vi "TRR_Main.vi"() -> ()   [LabVIEW 2020]
uses:
  Global 1.vi
panel:
  in  "Median Filter Rank":i32=5
  out "CURRENT RESULT":dbl[](array[numeric])
  in  "START TEST":bool
  out "Started":bool
  out "Elapsed time (minutes)":dbl
  out "start time":timestamp
  out "Oscilloscope Capture":waveform(dbl)[](graph)
  out "ALL RESULT Array":dbl[][](array[numeric])
  out "TEST#   |  Elapsed Time (minutes)":dbl[][](array[numeric])
  out "TRR :\nTotal Test Time (minutes)":dbl
  in  "Finish?":bool
  out "Cluster 3":T1
  out "Cluster 2":T2
  out "Cluster 1":T3
  in  "Cluster : Setting":T4={"VGE (V)"=0.0, "VCE (V)"=0.0, "ICE (A)"=0.0, "TEKTRONIX"="", "PROJECT #"="", "TEMPERATURE (C)"=0.0, "RG (Ohm)"=0.0, "DUT #"=1, "REQUEST #"="", "TEST #"=1}
  out "error out":errorcluster
  in  "error in (no error)":errorcluster
  # "PRODUCED BY : AFIQAH HASBULLAH ( SBN CZ ENG : 2022)"
  # "AC MODULE : TRR"
  # "Column 2"
  # "Column 3"
  # "Column 4"
  # "Column 5"
  # "Column 6"
  # "Column 7"
  # "Column 8"
  # "Column 9"
  # "Column 10"
  # "Column 0"
  # "Column 1"
  # "Column 11"
  # "Column 12"
  # "Column 13"
  # "Column 14"
  # "Column 15"
  # "Ta\n(ns)"
  # "Tb\n(ns)"
  # "Trr\n(ns)"
  # "Irrm\n(A)"
  # "Qrr\n(nC)"
  # "Erec\n(uJ)"
  # "Di/Dt\n(A/us)"
  # "Di\n(A)"
  # "Dt\n(us)"
  # "Vce"
  # "Ice"
  # "Vge"
  # "Rg"
  # "Temperature"
  # "DUT  #"
  # "TEST #"
  # "< Press 2 times >"
  # "Column 2"
  # "Column 3"
  # "Column 4"
  # "Column 5"
  # "Column 6"
  # "Column 7"
  # "Column 8"
  # "Column 9"
  # "Column 10"
  # "Column 0"
  # "Column 1"
  # "Column 11"
  # "Column 12"
  # "Column 13"
  # "Column 14"
  # "Column 15"
  # "Ta\n(ns)"
  # "Tb\n(ns)"
  # "Trr\n(ns)"
  # "Irrm\n(A)"
  # "Qrr\n(nC)"
  # "Erec\n(uJ)"
  # "Di/Dt\n(A/us)"
  # "Di\n(A)"
  # "Dt\n(us)"
  # "Vce"
  # "Ice"
  # "Vge"
  # "Rg"
  # "Temperature"
  # "DUT  #"
  # "TEST #"
  # "Done TRR & QRR Acquisition"
  # "Done Di/Dt Acquisition"
  # "Done Exporting image of Overall Waveform"
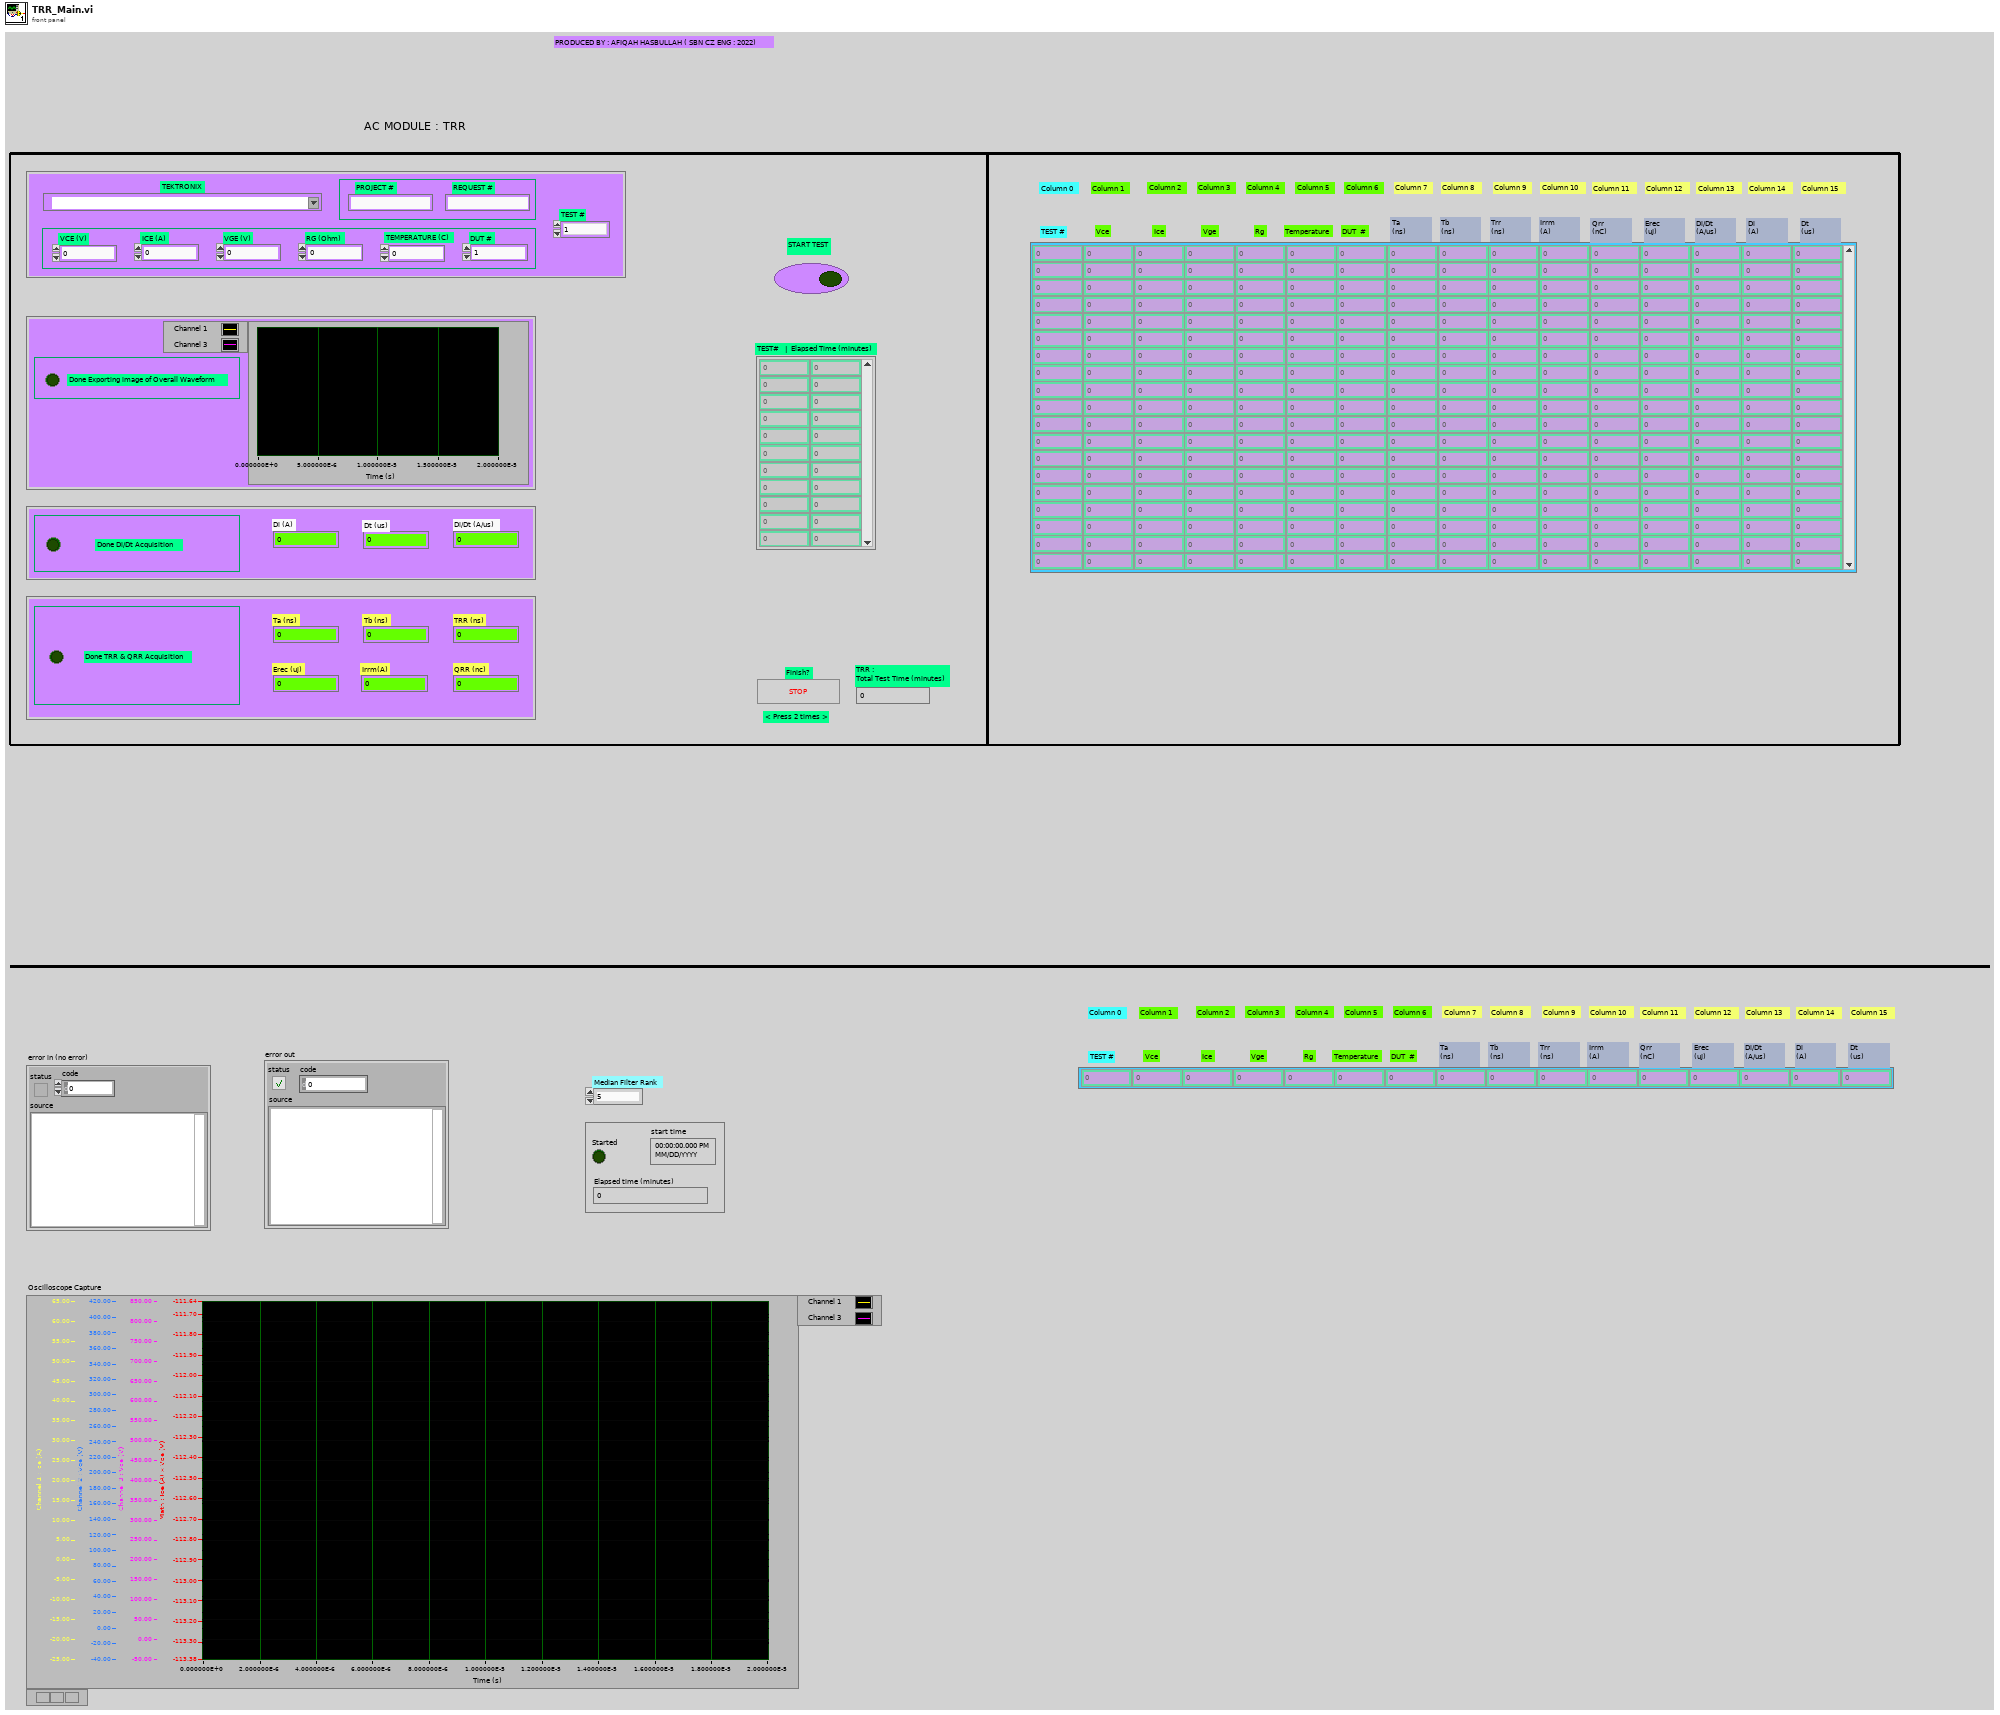
[diagram p1: front panel]
types:
  T1 = cluster{"Ta (ns)":dbl, "Tb (ns)":dbl, "Irrm(A)":dbl, "TRR (ns)":dbl, "QRR (nc)":dbl, "Erec (uj)":dbl, "LED 3":bool}
  T2 = cluster{"Di/Dt (A/us)":dbl, "Di (A)":dbl, "Dt (us)":dbl, "LED 2":bool}
  T3 = cluster{"LED 1":bool, "Oscilloscope Capture":waveform(dbl)[]}
  T4 = cluster{"VGE (V)":dbl, "VCE (V)":dbl, "ICE (A)":dbl, "TEKTRONIX":refnum<visa-resource-name>, "PROJECT #":string, "TEMPERATURE (C)":dbl, "RG (Ohm)":dbl, "DUT #":i32, "REQUEST #":string, "TEST #":i32}
  T5 = cluster{"Di/Dt (A/us)":dbl, "Di (A)":dbl, "Dt (ns)":dbl, "LED 2":bool}
  T6 = typedef "imagedata.ctl" = cluster{"image type":i32, "image depth":i32, "image":u8[], "mask":u8[], "colors":u32[], "Rectangle":cluster{"left":i16, "top":i16, "right":i16, "bottom":i16}}
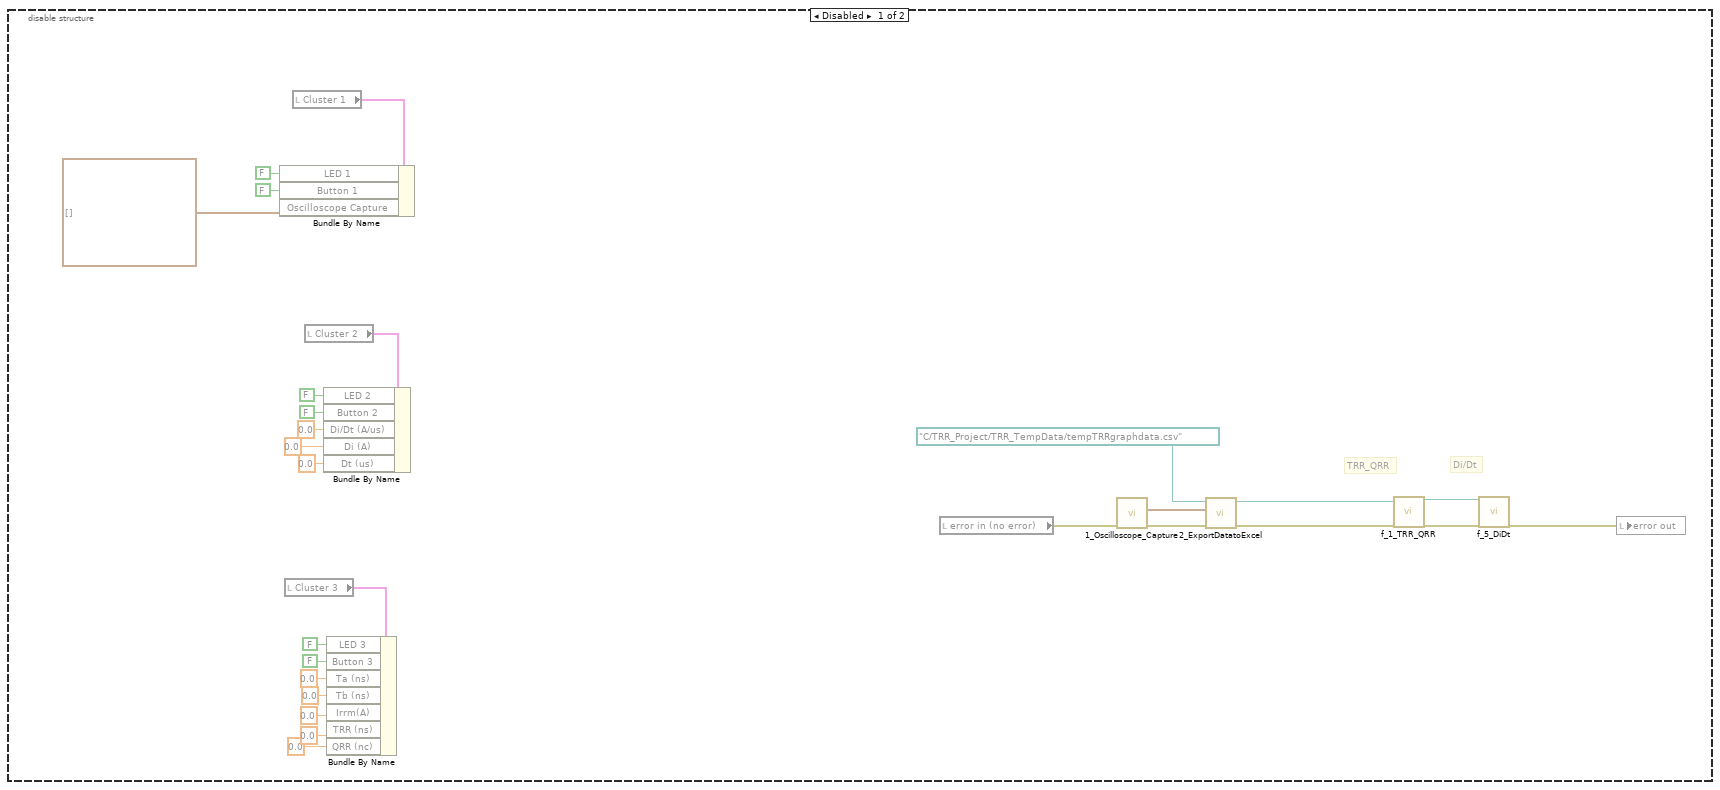
[diagram p3: hidden frame]
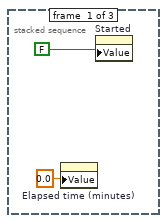
[diagram p4: hidden frame]
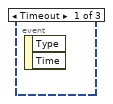
[diagram p6: hidden frame]
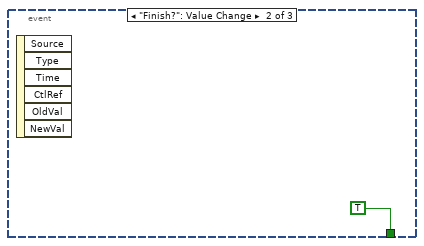
[diagram p7: hidden frame]
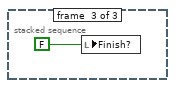
[diagram p9: hidden frame]
diagram:
  w1 = 5 ("Median Filter Rank")
  w17 = errorcluster {"status"=FALSE, "code"=0, "source"=""} ("error out")
  w4 = FALSE ("Started")
  w16 = 0.0 ("TRR :\nTotal Test Time (minutes)")
  n1 = flat-sequence {
    tunnel: [w27] -> w7
    tunnel: w7 -> [w28]
    tunnel: [w29] -> w6
    tunnel: w6 -> [w286]
    tunnel: [w281] -> w5
    tunnel: w5 -> [w312]
    frame #0 {
      # "IN"
      n2 = local read "error in (no error)"() -> (w27:errorcluster)
    }
    frame #1 {
      n3 = while {
        shift-right: [w32] -> w29
        shift-left: w28 -> [w31]
        stop <- w33 stop-if-true
        n4 = local read "START TEST"() -> (w35:bool)
        n5 = case shown="True" w35 {
          tunnel: w31 -> [w36 w53]
          tunnel: [w36 w46] -> w32
          frame False {
          }
          frame True {
            n6 = flat-sequence {
              tunnel: w53 -> [w60]
              tunnel: [w60] -> w45
              tunnel: w45 -> [w73]
              tunnel: [w73] -> w44
              tunnel: [w71] -> w43
              tunnel: [w70] -> w42
              tunnel: [w69] -> w41
              tunnel: [w68] -> w40
              tunnel: [w67] -> w39
              tunnel: [w66] -> w38
              tunnel: [w65] -> w37
              tunnel: w44 -> [w81]
              tunnel: [w81] -> w52
              tunnel: w43 -> [w80]
              tunnel: w42 -> [w79]
              tunnel: w41 -> [w78]
              tunnel: w40 -> [w77]
              tunnel: w39 -> [w76]
              tunnel: w38 -> [w75]
              tunnel: w37 -> [w74]
              tunnel: w52 -> [w108]
              tunnel: [w107] -> w51
              tunnel: w51 -> [w145]
              tunnel: [w141] -> w50
              tunnel: w50 -> [w196]
              tunnel: [w192] -> w49
              tunnel: w49 -> [w259]
              tunnel: [w259] -> w48
              tunnel: w48 -> [w267]
              tunnel: [w267] -> w47
              tunnel: w47 -> [w276]
              tunnel: [w276] -> w46
              frame #0 {
                # "Initialize"
                n7 = local read "Median Filter Rank"() -> (w54:i32)
                n8 = Initialize Array(0.0 ("element"), 16 ("dimension size")) -> (w57:dbl[])
                n9 = local write "Cluster 3"(T1 {"Ta (ns)"=0.0, "Tb (ns)"=0.0, "Irrm(A)"=0.0, "TRR (ns)"=0.0, "QRR (nc)"=0.0, "Erec (uj)"=0.0, "LED 3"=FALSE} ("Cluster 3")) -> ()
                n10 = global write "Global 1.vi" "Median Filter Rank"(w54) -> ()
                n11 = local write "Cluster 2"(T5 {"Di/Dt (A/us)"=0.0, "Di (A)"=0.0, "Dt (ns)"=0.0, "LED 2"=FALSE} ("Cluster 2")) -> ()
                n12 = local write "CURRENT RESULT"(w57) -> ()
                n13 = local write "Cluster 1"(T3 {"LED 1"=FALSE, "Oscilloscope Capture"=[]} ("Cluster 1")) -> ()
                n14 = local write "Oscilloscope Capture"(waveform(dbl)[] [] ("Oscilloscope Capture")) -> ()
                n15 = Wait (ms)(milliseconds to wait=u32 500) -> ()  [unwired: 1 out]
              }
              frame #1 {
                n16 = local read "Cluster : Setting"() -> (w72:T4)
                n17 = Unbundle By Name(w72) -> ("TEST #"=w71:i32, "VCE (V)"=w70:dbl, "ICE (A)"=w69:dbl, "VGE (V)"=w68:dbl, "RG (Ohm)"=w67:dbl, "TEMPERATURE (C)"=w66:dbl, "DUT #"=w65:i32)
                n18 = Wait (ms)(milliseconds to wait=u32 300) -> ()  [unwired: 1 out]
              }
              frame #2 {
                # "Column 6 = DUT#"
                # "Column 5 = Temperature"
                # "Column 4 = RG"
                # "Column 3 = VGE"
                # "Column 2 = ICE"
                # "Column 1 = VCE"
                # "Column 0 = TEST#"
                # "Insert Test Condition"
                n19 = Wait (ms)(milliseconds to wait=u32 300) -> ()  [unwired: 1 out]
                n20 = local read "CURRENT RESULT"() -> (w84:dbl[])
                n21 = local read "CURRENT RESULT"() -> (w86:dbl[])
                n22 = local read "CURRENT RESULT"() -> (w88:dbl[])
                n23 = local read "CURRENT RESULT"() -> (w89:dbl[])
                n24 = local read "CURRENT RESULT"() -> (w96:dbl[])
                n25 = local read "CURRENT RESULT"() -> (w92:dbl[])
                n26 = local read "CURRENT RESULT"() -> (w94:dbl[])
                n27 = Replace Array Subset(array=w96, new element=w80, index=0) -> (w95:dbl[])
                n28 = Replace Array Subset(array=w94, new element=w79, index=1) -> (w93:dbl[])
                n29 = Replace Array Subset(array=w92, new element=w78, index=2) -> (w91:dbl[])
                n30 = Replace Array Subset(array=w89, new element=w77, index=3) -> (w90:dbl[])
                n31 = Replace Array Subset(array=w84, new element=w74, index=6) -> (w83:dbl[])
                n32 = Replace Array Subset(array=w88, new element=w76, index=4) -> (w87:dbl[])
                n33 = Replace Array Subset(array=w86, new element=w75, index=5) -> (w85:dbl[])
                n34 = local write "CURRENT RESULT"(w95) -> ()
                n35 = local write "CURRENT RESULT"(w93) -> ()
                n36 = local write "CURRENT RESULT"(w91) -> ()
                n37 = local write "CURRENT RESULT"(w90) -> ()
                n38 = local write "CURRENT RESULT"(w87) -> ()
                n39 = local write "CURRENT RESULT"(w85) -> ()
                n40 = local write "CURRENT RESULT"(w83) -> ()
              }
              frame #3 {
                n41 = Wait (ms)(milliseconds to wait=u32 300) -> ()  [unwired: 1 out]
                n42 = flat-sequence {
                  tunnel: w108 -> [w115]
                  tunnel: [w110] -> w105
                  tunnel: [w120] -> w104
                  tunnel: w105 -> [w119]
                  tunnel: [w136] -> w107
                  tunnel: w104 -> [w136]
                  frame #0 {
                    n43 = local read "Cluster : Setting"() -> (w114:T4)
                    n44 = Unbundle By Name(w114) -> ("TEKTRONIX"=w113:refnum<visa-resource-name>)
                    n45 = call "1_Oscilloscope_Capture.vi"("error in (no error)"=w115, "VISA Resource Name"=w113) -> ("error out"=w111:errorcluster, "Waveform Graph"=w109:waveform(dbl)[])  [unwired: 7 in, 1 out]
                    n46 = local write "Oscilloscope Capture"(w109) -> ()
                    n47 = local read "Cluster 1"() -> (w118:T3)
                    n48 = Bundle By Name(cluster=w118, "Oscilloscope Capture"=w109) -> (w117:T3)
                    n49 = local write "Cluster 1"(w117) -> ()
                    n50 = Wait (ms)(milliseconds to wait=u32 300) -> ()  [unwired: 1 out]
                    n51 = call "2_ExportDatatoExcel.vi"("error in (no error)"=w111, "Waveform Graph"=w109, "file path (IN)"=path "C:/TRR_Project/TRR_TempData/tempFullWaveformgraphdata.csv") -> ("error out"=w110:errorcluster)  [unwired: 7 in, 1 out]
                  }
                  frame #1 {
                    w132 = "_"
                    n52 = local read "Cluster : Setting"() -> (w127:T4)
                    n53 = Unbundle By Name(w127) -> ("PROJECT #"=w124:string, "REQUEST #"=w123:string, "TEST #"=w126:i32)
                    n54 = invoke on="Oscilloscope Capture" class="WFGraph (strict)" method="Get Image"(error in=w119) -> (error out=w128:errorcluster, "image data"=w129:T6)  [unwired: 5 in, 4 out]
                    n55 = Format Value(format string="%d", value (0)=w126) -> (output string=w122:string)  [unwired: 1 in]
                    n56 = Concatenate Strings("C:\\TRR_Project\\TRR_Image\\" ("string"), w124, w132, w123, w132, w122, w132, "TRR_FullWaveform" ("string"), ".png" ("string")) -> (w135:string)
                    n57 = String To Path(string=w135) -> (path=w134:path)
                    n58 = call <vilib>:"Write PNG File.vi"("error in (no error)"=w128, "image data"=w129, "path to PNG file"=w134) -> ("error out"=w120:errorcluster)  [unwired: 7 in, 1 out]
                    n59 = Wait (ms)(milliseconds to wait=u32 300) -> ()  [unwired: 1 out]
                  }
                  frame #2 {
                    n60 = local read "Cluster 1"() -> (w140:T3)
                    n61 = Bundle By Name(cluster=w140, "LED 1"=TRUE) -> (w138:T3)
                    n62 = Wait (ms)(milliseconds to wait=u32 300) -> ()  [unwired: 1 out]
                    n63 = local write "Cluster 1"(w138) -> ()
                  }
                }
              }
              frame #4 {
                # "Step 1 : Di/Dt"
                n64 = Wait (ms)(milliseconds to wait=u32 300) -> ()  [unwired: 1 out]
                n65 = flat-sequence {
                  tunnel: w145 -> [w150]
                  tunnel: [w150] -> w144
                  tunnel: [w156] -> w149
                  tunnel: [w155] -> w148
                  tunnel: [w151] -> w147
                  tunnel: w144 -> [w153]
                  tunnel: [w152] -> w142
                  tunnel: w149 -> [w176]
                  tunnel: w148 -> [w175]
                  tunnel: w147 -> [w174]
                  tunnel: [w172] -> w143
                  tunnel: w142 -> [w172]
                  tunnel: w143 -> [w186]
                  tunnel: [w186] -> w141
                  frame #0 {
                  }
                  frame #1 {
                    # "Di/Dt"
                    n66 = local read "Cluster : Setting"() -> (w165:T4)
                    n67 = Unbundle By Name(w165) -> ("ICE (A)"=w160:dbl, "PROJECT #"=w163:string, "REQUEST #"=w162:string, "TEST #"=w166:i32, "TEKTRONIX"=w159:refnum<visa-resource-name>)
                    n68 = call "1_Oscilloscope_Capture.vi"("error in (no error)"=w153, "VISA Resource Name"=w159) -> ("error out"=w170:errorcluster, "Waveform Graph"=w171:waveform(dbl)[])  [unwired: 7 in, 1 out]
                    n69 = call "2_ExportDatatoExcel.vi"("error in (no error)"=w170, "Waveform Graph"=w171, "file path (IN)"=path "C:/TRR_Project/TRR_TempData/tempDiDtgraphdata.csv") -> ("error out"=w167:errorcluster, "file path (OUT)"=w168:path)  [unwired: 7 in]
                    n70 = Format Value(format string="%d", value (0)=w166) -> (output string=w161:string)  [unwired: 1 in]
                    n71 = call "f_5_DiDt.vi"("file path (IN)"=w168, "Project #"=w163, "Request #"=w162, "TEST #"=w161, "error in (no error)"=w167, "ICE"=w160) -> ("Dt (us)"=w151:dbl, "Di (A)"=w155:dbl, "Di/Dt (A/us)"=w156:dbl, "error out"=w152:errorcluster)  [unwired: 5 in, 5 out]
                    n72 = local read "Cluster 2"() -> (w158:T2)
                    n73 = Bundle By Name(cluster=w158, "Di/Dt (A/us)"=w156, "Di (A)"=w155, "Dt (us)"=w151) -> (w157:T2)
                    n74 = Wait (ms)(milliseconds to wait=u32 300) -> ()  [unwired: 1 out]
                    n75 = local write "Cluster 2"(w157) -> ()
                  }
                  frame #2 {
                    # "Column 15 = Dt"
                    # "Column 14 = Di"
                    # "Column 13 = DiDt"
                    n76 = local read "CURRENT RESULT"() -> (w180:dbl[])
                    n77 = local read "CURRENT RESULT"() -> (w178:dbl[])
                    n78 = local read "CURRENT RESULT"() -> (w182:dbl[])
                    n79 = Wait (ms)(milliseconds to wait=u32 300) -> ()  [unwired: 1 out]
                    n80 = Replace Array Subset(array=w178, new element=w174, index=15) -> (w177:dbl[])
                    n81 = Replace Array Subset(array=w180, new element=w175, index=14) -> (w179:dbl[])
                    n82 = Replace Array Subset(array=w182, new element=w176, index=13) -> (w181:dbl[])
                    n83 = local write "CURRENT RESULT"(w177) -> ()
                    n84 = local write "CURRENT RESULT"(w179) -> ()
                    n85 = local write "CURRENT RESULT"(w181) -> ()
                  }
                  frame #3 {
                    n86 = local read "Cluster 2"() -> (w189:T2)
                    n87 = Bundle By Name(cluster=w189, "LED 2"=TRUE ("LED 1")) -> (w190:T2)
                    n88 = Wait (ms)(milliseconds to wait=u32 300) -> ()  [unwired: 1 out]
                    n89 = local write "Cluster 2"(w190) -> ()
                  }
                }
              }
              frame #5 {
                # "Step 2 : Irrm, Ta, Tb, TRR, QRR, Erec"
                n90 = Wait (ms)(milliseconds to wait=u32 300) -> ()  [unwired: 1 out]
                n91 = flat-sequence {
                  tunnel: w196 -> [w203]
                  tunnel: [w203] -> w195
                  tunnel: [w211] -> w202
                  tunnel: [w210] -> w201
                  tunnel: [w209] -> w200
                  tunnel: [w208] -> w199
                  tunnel: [w207] -> w198
                  tunnel: [w206] -> w197
                  tunnel: w195 -> [w205]
                  tunnel: [w204] -> w193
                  tunnel: w202 -> [w234]
                  tunnel: w201 -> [w233]
                  tunnel: w200 -> [w232]
                  tunnel: w199 -> [w231]
                  tunnel: w198 -> [w230]
                  tunnel: w197 -> [w229]
                  tunnel: [w228] -> w194
                  tunnel: w193 -> [w228]
                  tunnel: w194 -> [w254]
                  tunnel: [w254] -> w192
                  frame #0 {
                  }
                  frame #1 {
                    # "TRR_QRR"
                    n92 = local read "Cluster : Setting"() -> (w223:T4)
                    n93 = Unbundle By Name(w223) -> ("ICE (A)"=w214:dbl, "PROJECT #"=w215:string, "REQUEST #"=w213:string, "TEST #"=w224:i32, "TEKTRONIX"=w221:refnum<visa-resource-name>)
                    n94 = call "1_Oscilloscope_Capture.vi"("error in (no error)"=w205, "VISA Resource Name"=w221) -> ("error out"=w226:errorcluster, "Waveform Graph"=w227:waveform(dbl)[])  [unwired: 7 in, 1 out]
                    n95 = call "2_ExportDatatoExcel.vi"("error in (no error)"=w226, "Waveform Graph"=w227, "file path (IN)"=path "C:/TRR_Project/TRR_TempData/tempTRRgraphdata.csv") -> ("error out"=w217:errorcluster, "file path (OUT)"=w216:path)  [unwired: 7 in]
                    n96 = Format Value(format string="%d", value (0)=w224) -> (output string=w212:string)  [unwired: 1 in]
                    n97 = call "f_1_TRR_QRR.vi"("file path (IN)"=w216, "Project #"=w215, "Request #"=w213, "TEST #"=w212, "error in (no error)"=w217, "ICE"=w214) -> ("Ta (ns)"=w211:dbl, "Tb (ns)"=w210:dbl, "Irrm(A)"=w208:dbl, "Erec (uj)"=w206:dbl, "TRR (ns)"=w209:dbl, "QRR (nc)"=w207:dbl, "error out"=w204:errorcluster)  [unwired: 5 in, 2 out]
                    n98 = local read "Cluster 3"() -> (w220:T1)
                    n99 = Bundle By Name(cluster=w220, "Ta (ns)"=w211, "Tb (ns)"=w210, "Irrm(A)"=w208, "TRR (ns)"=w209, "QRR (nc)"=w207, "Erec (uj)"=w206) -> (w219:T1)
                    n100 = local write "Cluster 3"(w219) -> ()
                    n101 = Wait (ms)(milliseconds to wait=u32 300) -> ()  [unwired: 1 out]
                  }
                  frame #2 {
                    # "Column 12 = Erec"
                    # "Column 11 = Qrr"
                    # "Column 10 = Irrm"
                    # "Column 9 = Trr"
                    # "Column 8 = Tb"
                    # "Column 7 = Ta"
                    n102 = local read "CURRENT RESULT"() -> (w248:dbl[])
                    n103 = local read "CURRENT RESULT"() -> (w246:dbl[])
                    n104 = local read "CURRENT RESULT"() -> (w250:dbl[])
                    n105 = local read "CURRENT RESULT"() -> (w240:dbl[])
                    n106 = local read "CURRENT RESULT"() -> (w242:dbl[])
                    n107 = local read "CURRENT RESULT"() -> (w238:dbl[])
                    n108 = Wait (ms)(milliseconds to wait=u32 300) -> ()  [unwired: 1 out]
                    n109 = Replace Array Subset(array=w246, new element=w232, index=9) -> (w245:dbl[])
                    n110 = Replace Array Subset(array=w248, new element=w233, index=8) -> (w247:dbl[])
                    n111 = Replace Array Subset(array=w250, new element=w234, index=7) -> (w249:dbl[])
                    n112 = Replace Array Subset(array=w242, new element=w229, index=12) -> (w243:dbl[])
                    n113 = Replace Array Subset(array=w240, new element=w230, index=11) -> (w241:dbl[])
                    n114 = Replace Array Subset(array=w238, new element=w231, index=10) -> (w239:dbl[])
                    n115 = local write "CURRENT RESULT"(w245) -> ()
                    n116 = local write "CURRENT RESULT"(w247) -> ()
                    n117 = local write "CURRENT RESULT"(w243) -> ()
                    n118 = local write "CURRENT RESULT"(w241) -> ()
                    n119 = local write "CURRENT RESULT"(w249) -> ()
                    n120 = local write "CURRENT RESULT"(w239) -> ()
                  }
                  frame #3 {
                    n121 = local read "Cluster 3"() -> (w257:T1)
                    n122 = Bundle By Name(cluster=w257, "LED 3"=TRUE ("LED 1")) -> (w258:T1)
                    n123 = Wait (ms)(milliseconds to wait=u32 300) -> ()  [unwired: 1 out]
                    n124 = local write "Cluster 3"(w258) -> ()
                  }
                }
              }
              frame #6 {
                # "Update Data in All Result Array"
                n125 = local read "Cluster : Setting"() -> (w266:T4)
                n126 = Unbundle By Name(w266) -> ("TEST #"=w264:i32)
                n127 = local read "CURRENT RESULT"() -> (w262:dbl[])
                n128 = local read "ALL RESULT Array"() -> (w263:dbl[][])
                n129 = Wait (ms)(milliseconds to wait=u32 300) -> ()  [unwired: 1 out]
                n130 = Decrement(x=w264) -> (x-1=w265:i32)
                n131 = Replace Array Subset(array=w263, new element=w262, index (row)=w265) -> (w261:dbl[][])  [unwired: 1 in]
                n132 = local write "ALL RESULT Array"(w261) -> ()
              }
              frame #7 {
                # "Increment TEST# & DUT#"
                n133 = local read "Cluster : Setting"() -> (w275:T4)
                n134 = Unbundle By Name(w275) -> ("TEST #"=w274:i32, "DUT #"=w273:i32)
                n135 = Increment(x=w274) -> (x+1=w270:i32)
                n136 = Increment(x=w273) -> (x+1=w269:i32)
                n137 = local read "Cluster : Setting"() -> (w272:T4)
                n138 = Wait (ms)(milliseconds to wait=u32 200) -> ()  [unwired: 1 out]
                n139 = Bundle By Name(cluster=w272, "TEST #"=w270, "DUT #"=w269) -> (w271:T4)
                n140 = local write "Cluster : Setting"(w271) -> ()
              }
              frame #8 {
                n141 = local write "START TEST"(FALSE ("START TEST")) -> ()
                n142 = local write "Started"(FALSE ("Started")) -> ()
                n143 = Wait (ms)(milliseconds to wait=u32 1000) -> ()  [unwired: 1 out]
              }
            }
          }
        }
        n144 = Wait (ms)(milliseconds to wait=u32 300) -> ()  [unwired: 1 out]
        n145 = local read "Finish?"() -> (w33:bool)
      }
      n146 = Wait (ms)(milliseconds to wait=u32 300) -> ()  [unwired: 1 out]
    }
    frame #2 {
      # "Minutes"
      # "Export to Excel"
      n147 = local read "Cluster : Setting"() -> (w295:T4)
      n148 = local read "TEST#   |  Elapsed Time (minutes)"() -> (w291:dbl[][])
      n149 = Unbundle By Name(w295) -> ("TEST #"=w292:i32)
      n150 = Index Array(array=w291, index (col)=1 ("disabled index (col)")) -> (element=w294:dbl[])  [unwired: 1 in]
      n151 = local read "ALL RESULT Array"() -> (w296:dbl[][])
      n152 = Decrement(x=w292) -> (x-1=w293:i32)
      n153 = Split 1D Array(array=w294, index=w293) -> (first subarray=w288:dbl[])  [unwired: 1 out]
      n154 = Decrement(x=w292) -> (x-1=w297:i32)
      n155 = local read "Cluster : Setting"() -> (w303:T4)
      n156 = for {
        tunnel: w288 -> [w311] mode=indexing
        shift-right: [w308] -> w287
        shift-left: 0.0 -> [w310]
        shift-right: [w309] -> w284
        shift-left: w286 -> [w309]
        n157 = Add(x=w311, y=w310) -> (x+y=w308:dbl)
        n158 = local write "TRR :\nTotal Test Time (minutes)"(w308) -> ()
      }
      n159 = Array Subset(array=w296, index (row)=0 ("index"), length (row)=w297, index (col)=0 ("index"), length (col)=16 ("length")) -> (w282:dbl[][])
      n160 = Unbundle By Name(w303) -> ("PROJECT #"=w302:string, "REQUEST #"=w301:string)
      n161 = call "O_Data_to_Excel.vi"("error in (no error)"=w286, "ALL RESULT Array"=w282, "REQUEST #"=w301, "PROJECT #"=w302) -> ("error out"=w283:errorcluster)  [unwired: 7 in]
      n162 = Wait (ms)(milliseconds to wait=u32 400) -> ()  [unwired: 1 out]
      n163 = local write "TRR :\nTotal Test Time (minutes)"(w287) -> ()
      n164 = Merge Errors(w283, w284) -> (w285:errorcluster)
      n165 = while {
        shift-right: [w304] -> w281
        shift-left: w285 -> [w305]
        stop <- w306 stop-if-true
        n166 = call "Display Message to User"("error in (no error)"=w305) -> ("error out"=w304:errorcluster, "OK"=w306:bool)  [unwired: 9 in]
        n167 = Wait (ms)(milliseconds to wait=u32 100) -> ()  [unwired: 1 out]
      }
    }
    frame #3 {
      # "OUT"
      n168 = local write "error out"(w312) -> ()
    }
  }
  n169 = local read "Cluster : Setting"() -> (w15:T4)
  n170 = Bundle By Name(cluster=w15, "TEST #"=1, "DUT #"=1) -> (w14:T4)
  n171 = local write "Cluster : Setting"(w14) -> ()
  n172 = Initialize Array(0.0 ("element"), 100 ("dimension size"), 2 ("dimension size")) -> (→"TEST#   |  Elapsed Time (minutes)":dbl[][])
  n173 = Initialize Array(0.0 ("element"), 100 ("dimension size"), 16 ("dimension size")) -> (→"ALL RESULT Array":dbl[][])
  n174 = Initialize Array(0.0 ("element"), 16 ("dimension size")) -> (→"CURRENT RESULT":dbl[])
  n175 = local write "Median Filter Rank"(w1) -> ()
  n176 = local write "START TEST"(w4) -> ()
  n177 = global write "Global 1.vi" "Median Filter Rank"(w1) -> ()
  n178 = local write "Started"(w4) -> ()
  n179 = local write "Finish?"(w4) -> ()
  n180 = local write "error out"(w17) -> ()
  n181 = local write "error in (no error)"(w17) -> ()
  n182 = disable-structure shown="Enabled" {
    frame Disabled {
      # "Di/Dt"
      # "TRR_QRR"
      n183 = local read "Cluster 3"() -> (w329:T1)
      n184 = local read "Cluster 1"() -> (w339:T3)
      n185 = Bundle By Name(cluster=w339, "LED 1"=FALSE, "Button 1"=FALSE, "Oscilloscope Capture"=waveform(dbl)[] []) -> ()  [unwired: 1 out]
      n186 = local read "Cluster 2"() -> (w338:T2)
      n187 = Bundle By Name(cluster=w338, "LED 2"=FALSE, "Button 2"=FALSE, "Di/Dt (A/us)"=0.0, "Di (A)"=0.0, "Dt (us)"=0.0 ("Dt (ns)")) -> ()  [unwired: 1 out]
      n188 = Bundle By Name(cluster=w329, "LED 3"=FALSE, "Button 3"=FALSE, "Ta (ns)"=0.0, "Tb (ns)"=0.0, "Irrm(A)"=0.0, "TRR (ns)"=0.0, "QRR (nc)"=0.0) -> ()  [unwired: 1 out]
      n189 = local read "error in (no error)"() -> (w320:errorcluster)
      n190 = call "1_Oscilloscope_Capture.vi"("error in (no error)"=w320) -> ("error out"=w314:errorcluster, "Waveform Graph"=w317:waveform(dbl)[])  [unwired: 8 in, 1 out]
      n191 = call "2_ExportDatatoExcel.vi"("error in (no error)"=w314, "Waveform Graph"=w317, "file path (IN)"=path "C:/TRR_Project/TRR_TempData/tempTRRgraphdata.csv") -> ("error out"=w316:errorcluster, "file path (OUT)"=w315:path)  [unwired: 7 in]
      n192 = call "f_1_TRR_QRR.vi"("file path (IN)"=w315, "error in (no error)"=w316) -> ("file path (OUT)"=w319:path, "error out"=w318:errorcluster)  [unwired: 9 in, 7 out]
      n193 = call "f_5_DiDt.vi"("file path (IN)"=w319, "error in (no error)"=w318) -> ("error out"=w321:errorcluster)  [unwired: 9 in, 8 out]
      n194 = local write "error out"(w321) -> ()
    }
    frame Enabled {
    }
  }
  n195 = while {
    stop <- w341 stop-if-true
    # "COPY from NI Forum :)"
    n196 = stacked-sequence {
      tunnel: [_ w344 _] -> w341
      frame #0 {
        n197 = property on="Elapsed time (minutes)" class="DigNum (strict)"("Value"=0.0 ("Elapsed time (seconds)")) -> ()  [unwired: 2 in, 2 out]
        n198 = property on="Started" class="Bool (strict)"("Value"=FALSE ("Started")) -> ()  [unwired: 2 in, 2 out]
      }
      frame #1 {
        n199 = while {
          tunnel: [w345] -> w344
          stop <- w345 stop-if-true
          n200 = local read "Started"() -> (w346:bool)
          n201 = case shown="True" w346 {
            frame False {
              # "do nothing"
            }
            frame True {
              n202 = local read "start time"() -> (w358:timestamp)
              n203 = local read "Cluster : Setting"() -> (w354:T4)
              n204 = Get Date/Time In Seconds() -> (seconds since 1Jan1904=w357:timestamp)
              n205 = Subtract(x=w357, y=w358) -> (x-y=w356:dbl)
              n206 = Divide(x=w356, y=60.0) -> (x/y=w348:dbl)
              n207 = Unbundle By Name(w354) -> ("TEST #"=w350:i32)
              n208 = local write "Elapsed time (minutes)"(w348) -> ()
              n209 = Build Array(w350, w348) -> (w351:dbl[])
              n210 = local read "TEST#   |  Elapsed Time (minutes)"() -> (w353:dbl[][])
              n211 = Decrement(x=w350) -> (x-1=w349:i32)
              n212 = Replace Array Subset(array=w353, new element=w351, index (row)=w349) -> (w352:dbl[][])  [unwired: 1 in]
              n213 = local write "TEST#   |  Elapsed Time (minutes)"(w352) -> ()
            }
          }
          n214 = local read "Finish?"() -> (w345:bool)
          n215 = Wait (ms)(milliseconds to wait=u32 10) -> ()  [unwired: 1 out]
        }
        n216 = while {
          stop <- w359 stop-if-true
          n217 = event shown="[2] \"START TEST\": Value Change" {
            selector: _ -> [_ _ _]
            dyn-events: _ -> [_ _ _]
            timeout: _ -> [_ _ _]
            tunnel: [_ TRUE FALSE] -> w359
            event Timeout {
              n218 = event-data() -> ()  [unwired: 1 in, 2 out]
            }
            event "Finish?": Value Change {
              n219 = event-data() -> ()  [unwired: 1 in, 6 out]
            }
            event "START TEST": Value Change {
              n220 = event-data() -> ()  [unwired: 1 in, 6 out]
              n221 = local read "Started"() -> (w363:bool)
              n222 = Not(x=w363) -> (.not. x?=w361:bool)
              n223 = case shown="True" w361 {
                frame False {
                }
                frame True {
                  n224 = Get Date/Time In Seconds() -> (seconds since 1Jan1904=→"start time":timestamp)
                }
              }
              n225 = local write "Started"(w361) -> ()
            }
          }
        }
      }
      frame #2 {
        n226 = local write "Finish?"(FALSE ("stop")) -> ()
      }
    }
    n227 = Wait (ms)(milliseconds to wait=u32 100) -> ()  [unwired: 1 out]
  }
  "Cluster 1" <- T3 {"LED 1"=FALSE, "Oscilloscope Capture"=[]} ("Cluster 1")
  "Cluster 2" <- T5 {"Di/Dt (A/us)"=0.0, "Di (A)"=0.0, "Dt (ns)"=0.0, "LED 2"=FALSE} ("Cluster 2")
  "Cluster 3" <- T1 {"Ta (ns)"=0.0, "Tb (ns)"=0.0, "Irrm(A)"=0.0, "TRR (ns)"=0.0, "QRR (nc)"=0.0, "Erec (uj)"=0.0, "LED 3"=FALSE} ("Cluster 3")
  "TRR :\nTotal Test Time (minutes)" <- w16
  "Oscilloscope Capture" <- waveform(dbl)[] [] ("Oscilloscope Capture")
  "Elapsed time (minutes)" <- w16
